vi "TRITON_HRANGE_COMMAND.vi"(1 "Heater Range [A]":dbl, 2 "Temperature Control Channel":i32=5) -> (0 "Command String":string)   [LabVIEW 2009]
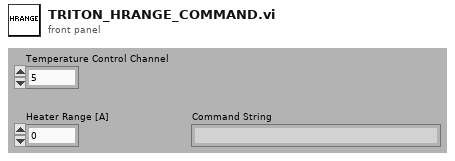
[diagram p1: front panel]
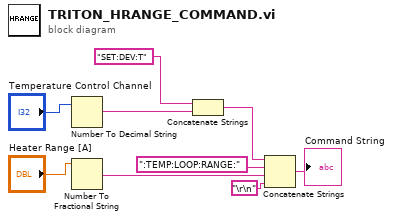
[diagram p0: block diagram]
diagram:
  n1 = Number To Decimal String(number="Temperature Control Channel") -> (decimal integer string=w6:string)  [unwired: 1 in]
  n2 = Number To Fractional String(number="Heater Range [A]") -> (F-format string=w3:string)  [unwired: 3 in]
  n3 = Concatenate Strings("SET:DEV:T", w6) -> (w5:string)
  n4 = Concatenate Strings(w5, ":TEMP:LOOP:RANGE:", w3, "\r\n") -> (→"Command String":string)
